vi "Project Path Setter.vi"(0 "ProjectPath In":path, 11 "error in (no error)":errorcluster) -> (15 "error out":errorcluster)   [LabVIEW 2021, in "Dictionary.lvlib"]
uses:
  Dictionary.lvlib
  controls/Dictionary States.ctl
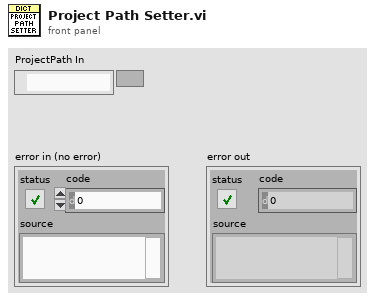
[diagram p1: front panel]
types:
  T1 = typedef "Dictionary.lvlib/Dictionary States.ctl" = enum16{"Set", "Get", "Delete", "Delete All"}
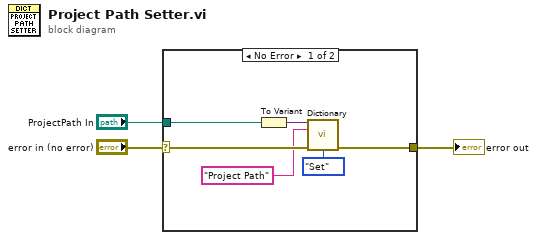
[diagram p0: block diagram]
diagram:
  n1 = case shown="No Error" "error in (no error)" {
    selector: "error in (no error)" -> [w8 w10]
    tunnel: [w7 w10] -> w2
    tunnel: "ProjectPath In" -> [w4 _]
    frame No Error {
      n2 = To Variant(anything=w4) -> (Variant=w6:variant)
      n3 = call "Dictionary.vi"("Variant_In"=w6, "Key"="Project Path", "error in (no error)"=w8, "Dictionary States"=Dictionary_States."Set" ("Dict States")) -> ("error out"=w7:errorcluster)  [unwired: 10 in, 1 out]
    }
    frame Error {
    }
  }
  "error out" <- w2
